vi "EEPROM Write.vi"   [LabVIEW 2014]
uses:
  QwaveSys_ESP8266/QwaveSys_ESP8266.lvlib
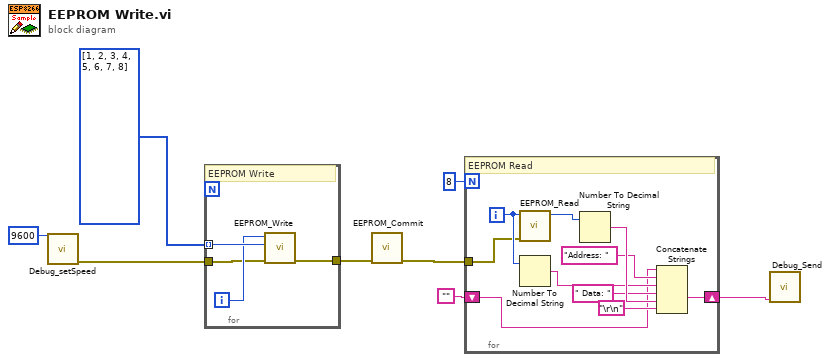
[diagram p0: block diagram]
diagram:
  n1 = call "Debug_setSpeed.vi"("Speed"=u32 9600) -> ("error out"=w2:errorcluster)  [unwired: 10 in]
  n2 = for {
    tunnel: u8[] [1, 2, 3, 4, 5, 6, 7, 8] ("Data") -> [w12] mode=indexing
    tunnel: [w10] -> w7
    tunnel: w2 -> [w9]
    i -> [w11]
    # "EEPROM Write"
    n3 = call "EEPROM_Write.vi"("error in (no error)"=w9, "Data"=w12, "Address"=w11) -> ("error out"=w10:errorcluster)  [unwired: 8 in]
  }
  n4 = call "EEPROM_Commit.vi"("error in (no error)"=w7) -> ("error out"=w6:errorcluster)  [unwired: 10 in]
  n5 = for {
    N: 8 -> [_]
    tunnel: w6 -> [w13]
    shift-right: [w20] -> w1
    shift-left: "" -> [w14]
    i -> [w18]
    # "EEPROM Read"
    n6 = call "EEPROM_Read.vi"("error in (no error)"=w13, "Address"=w18) -> ("Data"=w22:u8)  [unwired: 8 in, 1 out]
    n7 = Number To Decimal String(number=w18) -> (decimal integer string=w17:string)  [unwired: 1 in]
    n8 = Number To Decimal String(number=w22) -> (decimal integer string=w21:string)  [unwired: 1 in]
    n9 = Concatenate Strings(w14, "Address: " ("string"), w17, " Data: " ("string"), w21, "\r\n") -> (w20:string)
  }
  n10 = call "Debug_Send.vi"("DATA"=w1) -> ()  [unwired: 11 in]
